vi "Receive.vi"(8 "error in (no error)":errorcluster, 11 "VISA resource name":refnum<visa-resource-name>) -> (0 "error out":errorcluster, 3 "VISA resource name out":refnum<visa-resource-name>)   [LabVIEW 2013]
panel:
  out "Data":string
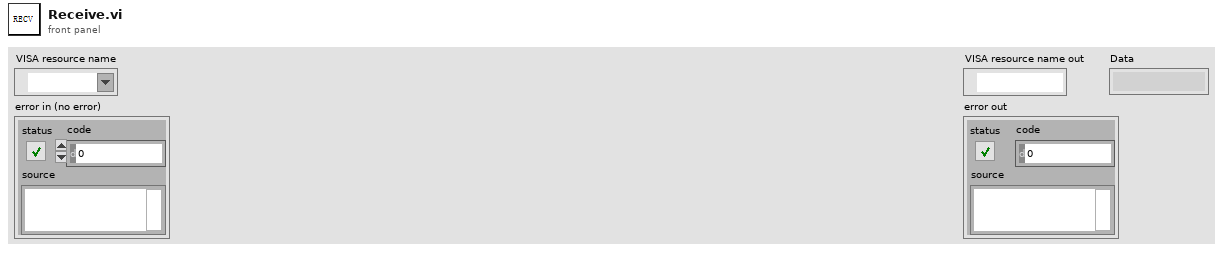
[diagram p1: front panel]
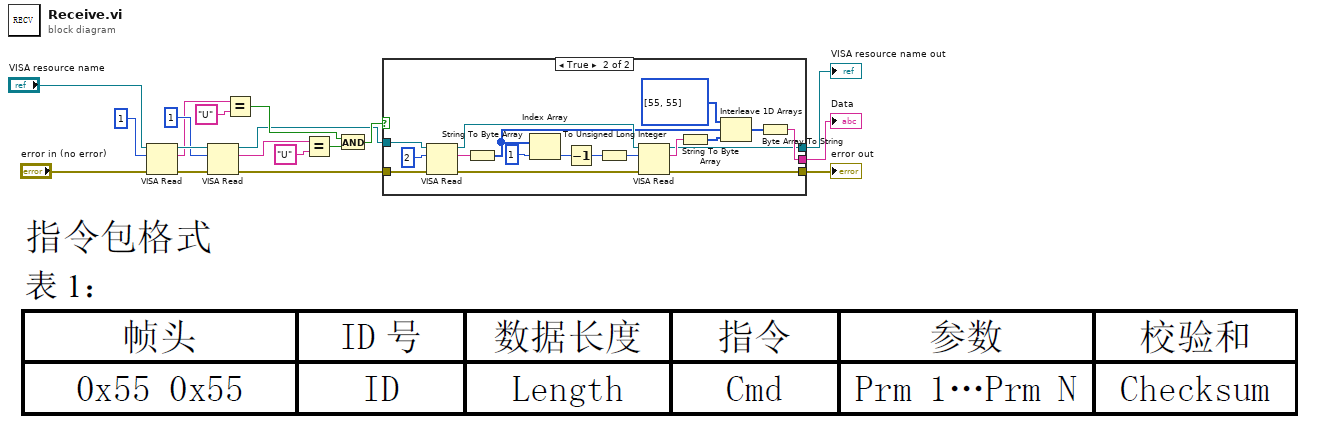
[diagram p0: block diagram]
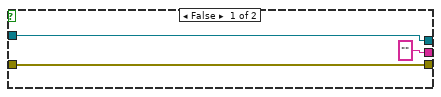
[diagram p2: hidden frame]
diagram:
  n1 = VISA Read(VISA resource name="VISA resource name", byte count=u32 1, error in (no error)="error in (no error)") -> (VISA resource name out=w15:refnum<visa-resource-name>, read buffer=w12:string, error out=w14:errorcluster)  [unwired: 1 out]
  n2 = VISA Read(VISA resource name=w15, byte count=u32 1, error in (no error)=w14) -> (VISA resource name out=w5:refnum<visa-resource-name>, read buffer=w11:string, error out=w4:errorcluster)  [unwired: 1 out]
  n3 = Equal?(x=w12, y="U") -> (x = y?=w7:bool)
  n4 = Equal?(x=w11, y="U") -> (x = y?=w8:bool)
  n5 = And(x=w7, y=w8) -> (x .and. y?=w6:bool)
  n6 = case shown="True" w6 {
    tunnel: w5 -> [w20 w39]
    tunnel: w4 -> [w19 w38]
    tunnel: ["" ("string") w25] -> w3
    tunnel: [w19 w23] -> w2
    tunnel: [w20 w22] -> w1
    frame False {
    }
    frame True {
      n7 = VISA Read(VISA resource name=w39, byte count=u32 2, error in (no error)=w38) -> (VISA resource name out=w32:refnum<visa-resource-name>, read buffer=w36:string, error out=w33:errorcluster)  [unwired: 1 out]
      n8 = String To Byte Array(string=w36) -> (unsigned byte array=w28:u8[])
      n9 = Index Array(array=w28, index=1) -> (element=w34:u8)
      n10 = Decrement(x=w34) -> (x-1=w31:u8)
      n11 = To Unsigned Long Integer(number=w31) -> (unsigned 32bit integer=w30:u32)
      n12 = VISA Read(VISA resource name=w32, byte count=w30, error in (no error)=w33) -> (VISA resource name out=w22:refnum<visa-resource-name>, read buffer=w29:string, error out=w23:errorcluster)  [unwired: 1 out]
      n13 = String To Byte Array(string=w29) -> (unsigned byte array=w27:u8[])
      n14 = Interleave 1D Arrays(u8[] [55, 55] ("array"), w28, w27) -> (w26:u8[])
      n15 = Byte Array To String(unsigned byte array=w26) -> (string=w25:string)
    }
  }
  "VISA resource name out" <- w1
  "error out" <- w2
  "Data" <- w3
